vi "Fpga-Exercisor-Top.vi"() -> ()   [LabVIEW 2017]
uses:
  <vilib>/Platform/TimedLoop/XDataNode/timing_clust.ctl
  <vilib>/Platform/TimedLoop/XDataNode/nitl_modes.ctl
  <vilib>/Platform/TimedLoop/XDataNode/wakeup.ctl
  <vilib>/rvi/Emulation/niFpgaSctlEmulationGetInTimedLoop.vi
  <vilib>/rvi/Emulation/niFpgaEmulationReportErrorSimple.vi
  <vilib>/rvi/Emulation/niFpgaGetClockAttributes.vi
  <vilib>/rvi/Emulation/niFpgaCriticalErrorInLSC.vi
  <vilib>/rvi/eio/common/nirviEmuTemplateMethod_errors.vi
  <vilib>/rvi/interface/RandomDataEmulation/niFpgaRandomDataHandleErrors.vi
  <vilib>/Platform/TimedLoop/XDataNode/XDataNode.xnode
  <vilib>/eio/EIONode/EIONode.xnode
  <vilib>/rvi/DataTransferAndStorage/Container/XNode/niFpgaContainer.xnode
  <vilib>/rvi/interface/RandomDataEmulation/nirviRandomDataFpgaReadWriteTemplate.vi
  <vilib>/Platform/TimedLoop/XDataNode/XDNodeRunTimeDep.lvlib
panel:
  out "AXI_STR_RXD_tready 2":bool
  out "tvalid 2":bool
  out "tdata 2":u32
  out "tlast 2":bool
  out "AXI_STR_RXD_tready_Count 2":u16
  out "tvalid_Count 2":u16
  out "tlast_Count 2":u16
  out "tdata_LastNonZero 2":u32
  out "AXI_STR_RXD_tready":bool
  out "tvalid":bool
  out "tdata":u32
  out "tlast":bool
  out "AXI_STR_RXD_tready_Count":u16
  out "tvalid_Count":u16
  out "tlast_Count":u16
  out "tdata_LastNonZero":u32
  out "d_microblaze\\gpio2_out_tri_o":u32
  in  "d_microblaze\\gpio2_in_tri_i":u32
  out "d_microblaze\\gpio1_out_tri_o":u32
  in  "d_microblaze\\gpio1_in_tri_i":u32
  in  "d_microblaze\\Int_1":bool
  in  "d_microblaze\\Int_0":bool
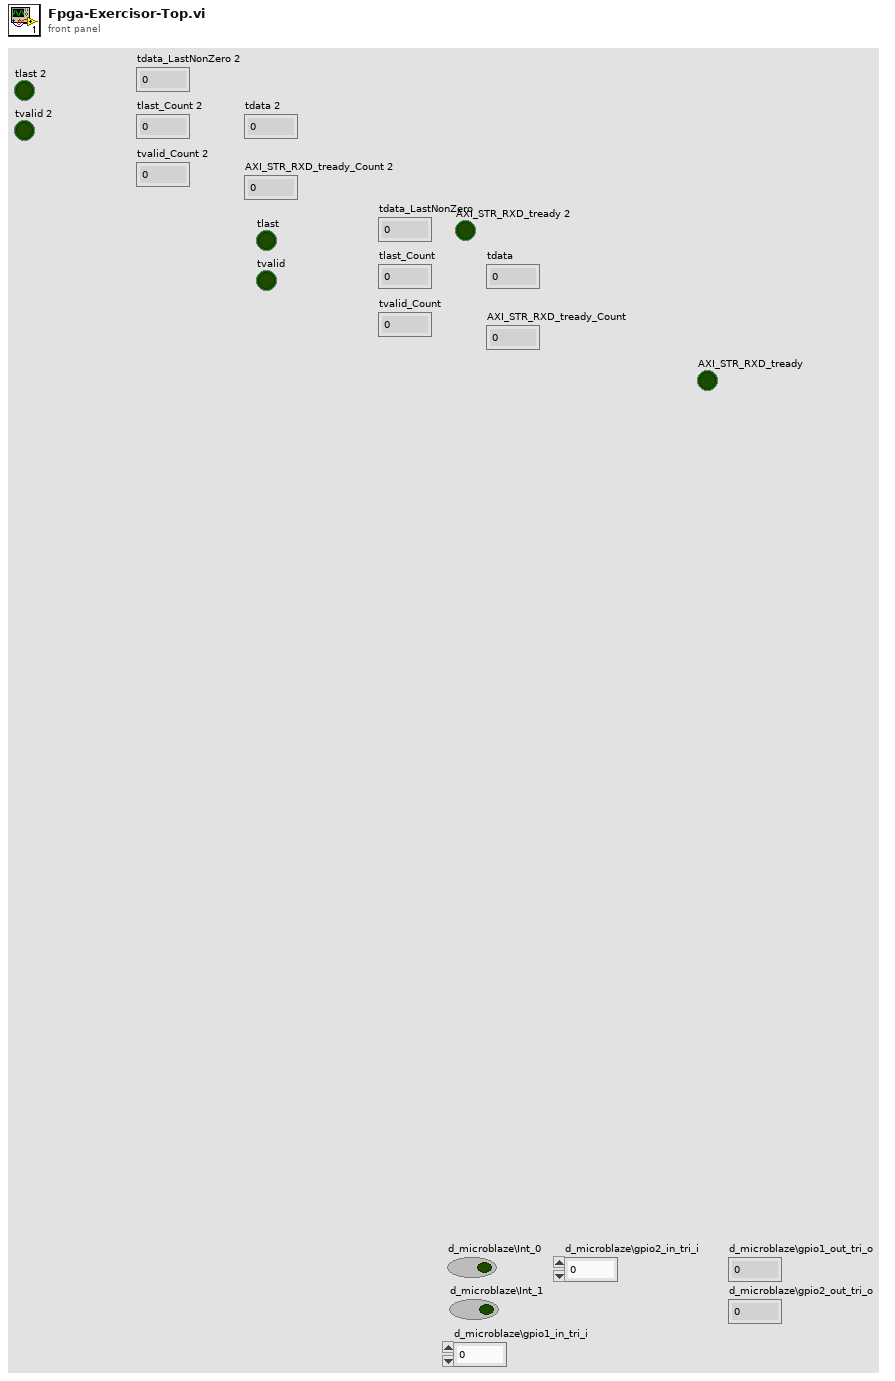
[diagram p1: front panel]
types:
  T1 = typedef "XDNodeRunTimeDep.lvlib/timing_clust.ctl" = cluster{"Expected End [f-1]":u64, "Actual End [f-1]":u64, "Finished Late? [f-1]":bool, "Expected End [i-1]":u64, "Actual End [i-1]":u64, "Finished Late? [i-1]":bool, "Expected Start [i]":u64, "Actual Start [i]":u64, "Expected Start [f]":u64, "Actual Start [f]":u64, "Source Name":string, "Structure Name":string, "Period":i64, "Deadline":i64, "Offset":i64, "Start":i64, "Priority":i32, "Timeout":i32, "Mode":T2, "Wakeup Reason":T3, "Error":errorcluster, "Source Type":string, "Secondary Source Type":string, "Global End Time":u64, "Global Start Time":u64, "Frame Duration":u64, "Iteration Duration":u64, "Assigned CPU":i32, "I/O Scan Engine Mode":u32}
  T2 = typedef "XDNodeRunTimeDep.lvlib/nitl_modes.ctl" = enum32{"No Change", "Process missed periods, maintain original phase", "Discard missed periods, maintain original phase", "Process missed periods, ignore original phase", "Discard missed periods, ignore original phase"}
  T3 = typedef "XDNodeRunTimeDep.lvlib/wakeup.ctl" = enum32{"Normal", "Aborted", "Asynchronous wakeup", "Timing source error", "Timed loop error", "Timeout"}
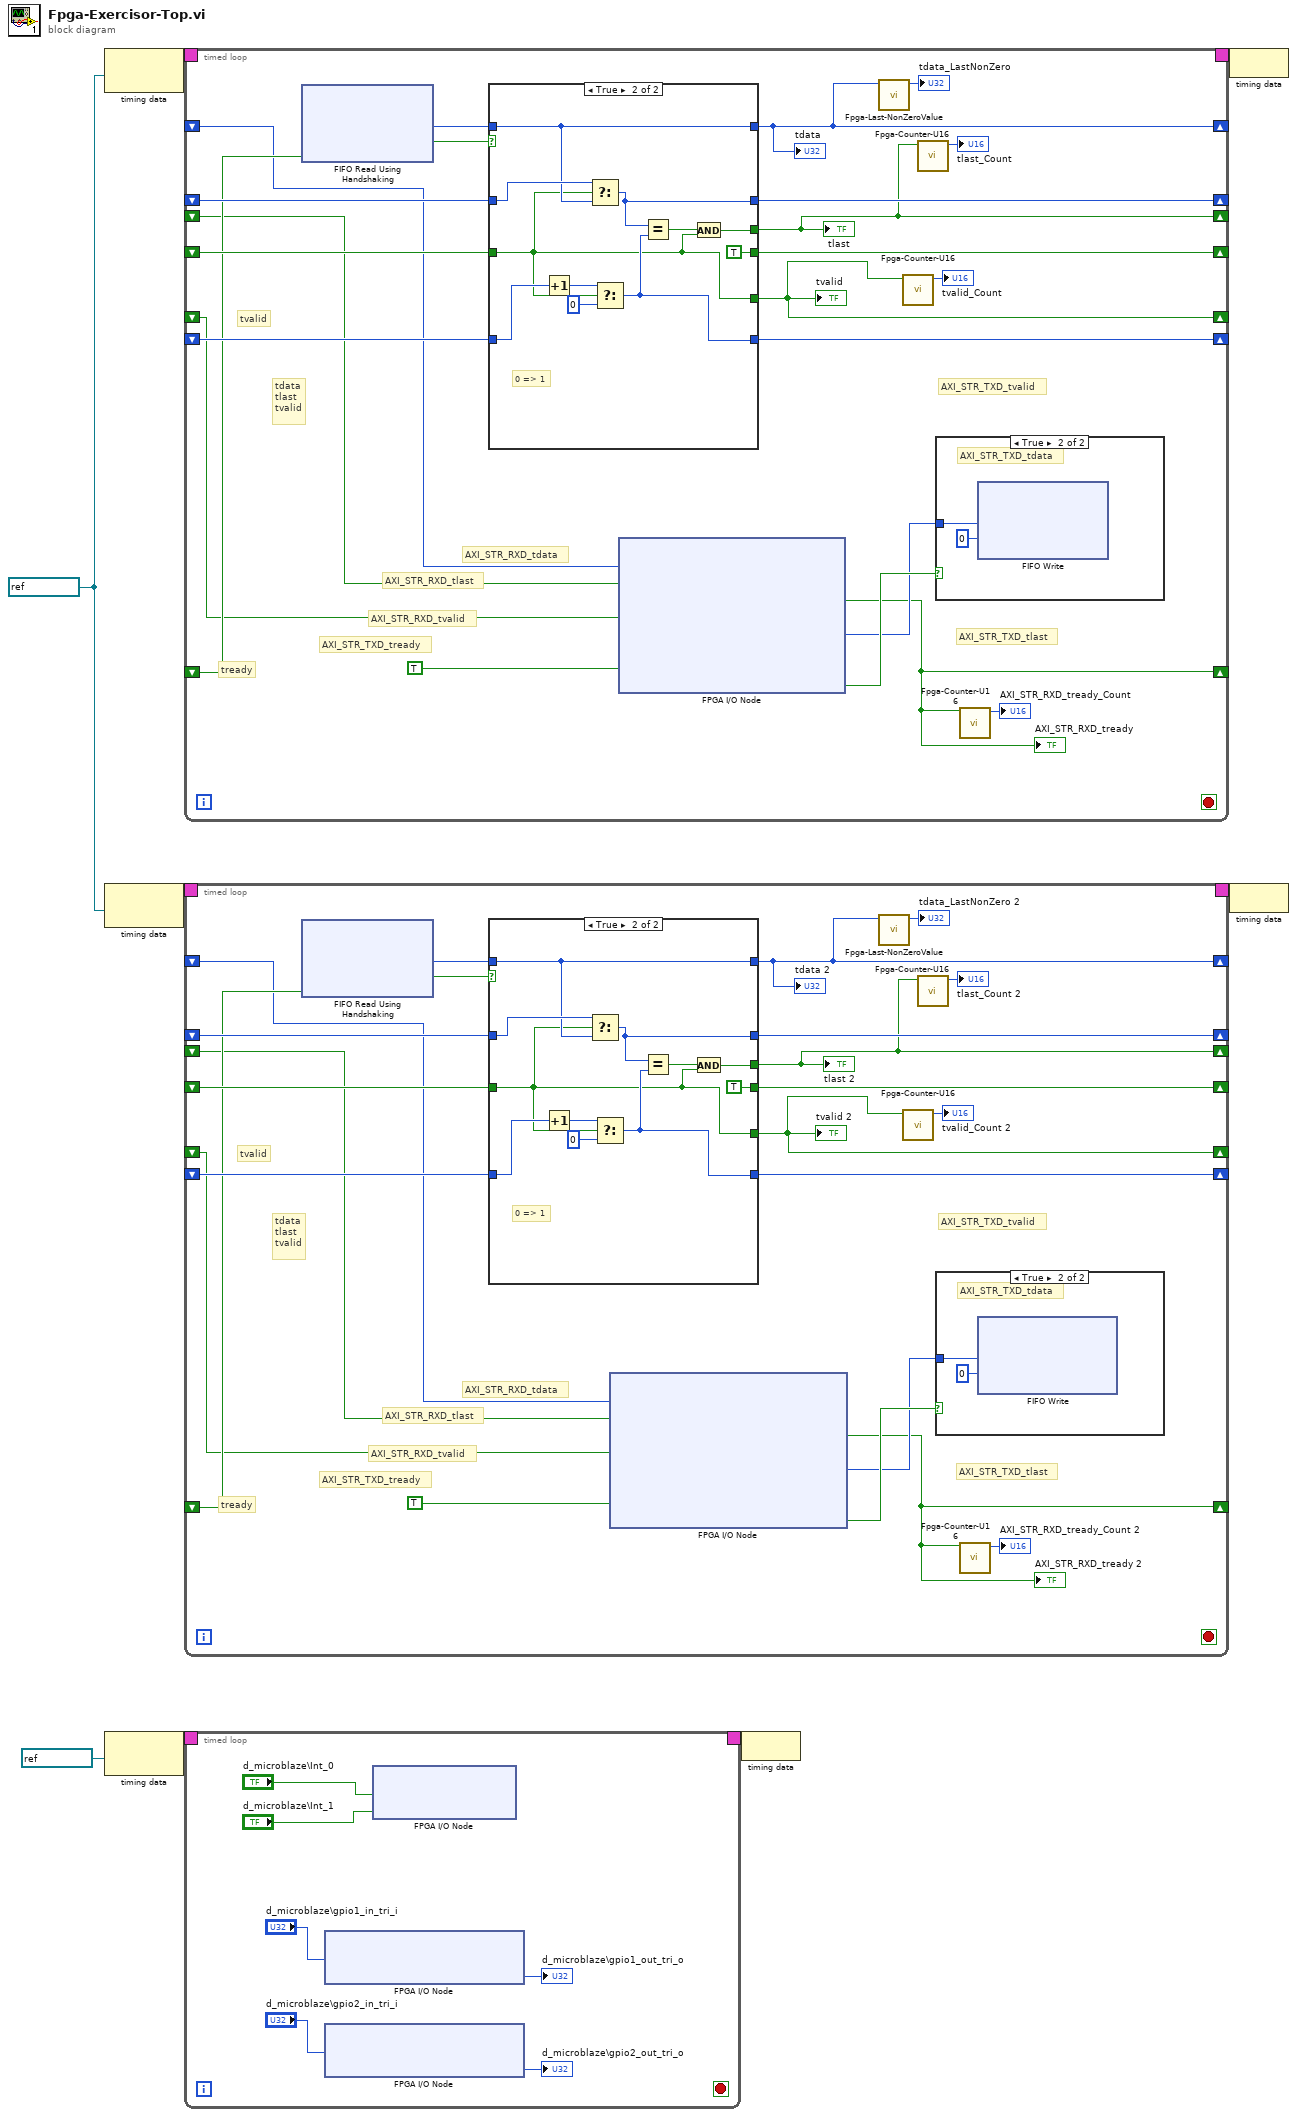
[diagram p0: block diagram]
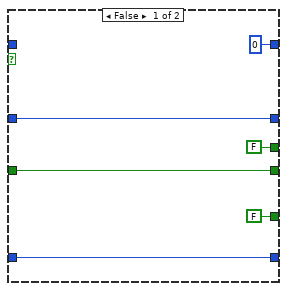
[diagram p3: hidden frame]
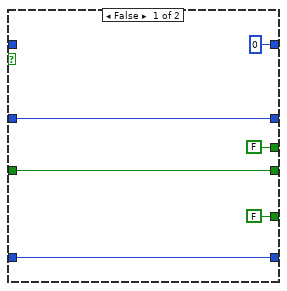
[diagram p5: hidden frame]
diagram:
  w1 = refnum<k21> "100MHz" ("Source Name")
  n1 = node-c288(w1) -> (w5:T1)
  n2 = node-c288(w1) -> (w3:T1)
  n3 = node-c288(refnum<k21> "100MHz" ("Source Name")) -> (w8:T1)
  n4 = timed-loop {
    timing: w5 -> [_]
    timing-out: [_] -> w4
    shift-right: [w29] -> _
    shift-left: _ -> [w30]
    shift-right: [w26] -> _
    shift-left: _ -> [w28]
    shift-right: [w24] -> _
    shift-left: _ -> [w25]
    shift-right: [w21] -> _
    shift-left: _ -> [w13]
    shift-right: [w9] -> _
    shift-left: _ -> [w23]
    shift-right: [w17] -> _
    shift-left: _ -> [w15]
    shift-right: [w19] -> _
    shift-left: _ -> [w14]
    stop <- _ stop-if-true
    # "AXI_STR_TXD_tlast"
    # "AXI_STR_TXD_tvalid"
    # "AXI_STR_TXD_tready"
    # "AXI_STR_RXD_tvalid"
    # "AXI_STR_RXD_tlast"
    # "AXI_STR_RXD_tdata"
    # "tvalid"
    # "tready"
    # "tdata\ntlast\ntvalid"
    n5 = xnode ("FIFO Read Using Handshaking")("Ready for Output"=w23) -> ("Element"=w27:u32, "Output Valid"=w31:bool)  [unwired: 1 in, 1 out]
    n6 = case shown="True" w31 {
      tunnel: w30 -> [w38 w40]
      tunnel: [w38 TRUE ("Size\nRead?")] -> w29
      tunnel: w28 -> [w39 w50]
      tunnel: w27 -> [_ w45]
      tunnel: [w39 w44] -> w26
      tunnel: w25 -> [w37 w49]
      tunnel: [w37 w43] -> w24
      tunnel: [FALSE ("Size\nRead?") w40] -> w21
      tunnel: [u32 0 ("Element") w45] -> w17
      tunnel: [FALSE w41] -> w19
      frame False {
      }
      frame True {
        # "0 => 1"
        n7 = Increment(x=w49) -> (x+1=w47:u32)
        n8 = Select(t=w50, s=w40, f=w45) -> (s? t:f=w44:u32)
        n9 = Select(t=w47, s=w40, f=u32 0) -> (s? t:f=w43:u32)
        n10 = Equal?(x=w44, y=w43) -> (x = y?=w42:bool)
        n11 = And(x=w42, y=w40) -> (x .and. y?=w41:bool)
      }
    }
    "tvalid" <- w21
    "tdata" <- w17
    "tlast" <- w19
    n12 = xnode "FPGA I/O Node"("d_microblaze\\AXI_STR_RXD_tdata"=w15, "d_microblaze\\AXI_STR_RXD_tlast"=w14, "d_microblaze\\AXI_STR_RXD_tvalid"=w13, "d_microblaze\\AXI_STR_TXD_tready"=TRUE ("d_microblaze\\AXI_STR_TXD_tready")) -> ("d_microblaze\\AXI_STR_RXD_tready"=w9:bool, "d_microblaze\\AXI_STR_TXD_tdata"=w10:u32, "d_microblaze\\AXI_STR_TXD_tvalid"=w11:bool)  [unwired: 8 in, 9 out]
    "AXI_STR_RXD_tready" <- w9
    n13 = call "Fpga-Last-NonZeroValue.vi"("d_mcs_i\\IO_BUS_write_data in"=w17) -> ("d_mcs_i\\IO_BUS_write_data out"=→"tdata_LastNonZero":u32)  [unwired: 10 in]
    n14 = call "Fpga-Counter-U16.vi"("d_mcs_i\\IO_BUS_read_strobe"=w21) -> ("Numeric"=→"tvalid_Count":u16)  [unwired: 10 in]
    n15 = call "Fpga-Counter-U16.vi"("d_mcs_i\\IO_BUS_read_strobe"=w19) -> ("Numeric"=→"tlast_Count":u16)  [unwired: 10 in]
    n16 = case shown="True" w11 {
      tunnel: w10 -> [_ w33]
      frame False {
      }
      frame True {
        # "AXI_STR_TXD_tdata"
        n17 = xnode ("FIFO Write")("Element"=w33, "Timeout"=0) -> ()  [unwired: 1 in, 2 out]
      }
    }
    n18 = call "Fpga-Counter-U16.vi"("d_mcs_i\\IO_BUS_read_strobe"=w9) -> ("Numeric"=→"AXI_STR_RXD_tready_Count":u16)  [unwired: 10 in]
  }
  n19 = timed-loop {
    timing: w3 -> [_]
    timing-out: [_] -> w2
    shift-right: [w73] -> _
    shift-left: _ -> [w74]
    shift-right: [w70] -> _
    shift-left: _ -> [w72]
    shift-right: [w68] -> _
    shift-left: _ -> [w69]
    shift-right: [w65] -> _
    shift-left: _ -> [w57]
    shift-right: [w53] -> _
    shift-left: _ -> [w67]
    shift-right: [w61] -> _
    shift-left: _ -> [w59]
    shift-right: [w63] -> _
    shift-left: _ -> [w58]
    stop <- _ stop-if-true
    # "AXI_STR_TXD_tlast"
    # "AXI_STR_TXD_tvalid"
    # "AXI_STR_TXD_tready"
    # "AXI_STR_RXD_tvalid"
    # "AXI_STR_RXD_tlast"
    # "AXI_STR_RXD_tdata"
    # "tvalid"
    # "tready"
    # "tdata\ntlast\ntvalid"
    n20 = xnode ("FIFO Read Using Handshaking")("Ready for Output"=w67) -> ("Element"=w71:u32, "Output Valid"=w75:bool)  [unwired: 1 in, 1 out]
    n21 = case shown="True" w75 {
      tunnel: w74 -> [w82 w84]
      tunnel: [w82 TRUE ("Size\nRead?")] -> w73
      tunnel: w72 -> [w83 w94]
      tunnel: w71 -> [_ w89]
      tunnel: [w83 w88] -> w70
      tunnel: w69 -> [w81 w93]
      tunnel: [w81 w87] -> w68
      tunnel: [FALSE ("Size\nRead?") w84] -> w65
      tunnel: [u32 0 ("Element") w89] -> w61
      tunnel: [FALSE w85] -> w63
      frame False {
      }
      frame True {
        # "0 => 1"
        n22 = Increment(x=w93) -> (x+1=w91:u32)
        n23 = Select(t=w94, s=w84, f=w89) -> (s? t:f=w88:u32)
        n24 = Select(t=w91, s=w84, f=u32 0) -> (s? t:f=w87:u32)
        n25 = Equal?(x=w88, y=w87) -> (x = y?=w86:bool)
        n26 = And(x=w86, y=w84) -> (x .and. y?=w85:bool)
      }
    }
    "tvalid 2" <- w65
    "tdata 2" <- w61
    "tlast 2" <- w63
    n27 = xnode "FPGA I/O Node"("d_microblaze\\AXI_STR_RXD_1_tdata"=w59, "d_microblaze\\AXI_STR_RXD_1_tlast"=w58, "d_microblaze\\AXI_STR_RXD_1_tvalid"=w57, "d_microblaze\\AXI_STR_TXD_1_tready"=TRUE ("d_microblaze\\AXI_STR_TXD_tready")) -> ("d_microblaze\\AXI_STR_RXD_1_tready"=w53:bool, "d_microblaze\\AXI_STR_TXD_1_tdata"=w54:u32, "d_microblaze\\AXI_STR_TXD_1_tvalid"=w55:bool)  [unwired: 8 in, 9 out]
    "AXI_STR_RXD_tready 2" <- w53
    n28 = call "Fpga-Last-NonZeroValue.vi"("d_mcs_i\\IO_BUS_write_data in"=w61) -> ("d_mcs_i\\IO_BUS_write_data out"=→"tdata_LastNonZero 2":u32)  [unwired: 10 in]
    n29 = call "Fpga-Counter-U16.vi"("d_mcs_i\\IO_BUS_read_strobe"=w65) -> ("Numeric"=→"tvalid_Count 2":u16)  [unwired: 10 in]
    n30 = call "Fpga-Counter-U16.vi"("d_mcs_i\\IO_BUS_read_strobe"=w63) -> ("Numeric"=→"tlast_Count 2":u16)  [unwired: 10 in]
    n31 = case shown="True" w55 {
      tunnel: w54 -> [_ w77]
      frame False {
      }
      frame True {
        # "AXI_STR_TXD_tdata"
        n32 = xnode ("FIFO Write")("Element"=w77, "Timeout"=0) -> ()  [unwired: 1 in, 2 out]
      }
    }
    n33 = call "Fpga-Counter-U16.vi"("d_mcs_i\\IO_BUS_read_strobe"=w53) -> ("Numeric"=→"AXI_STR_RXD_tready_Count 2":u16)  [unwired: 10 in]
  }
  n34 = timed-loop {
    timing: w8 -> [_]
    timing-out: [_] -> w7
    stop <- _ stop-if-true
    n35 = xnode "FPGA I/O Node"("d_microblaze\\gpio1_in_tri_i"="d_microblaze\\gpio1_in_tri_i") -> ("d_microblaze\\gpio1_out_tri_o"=→"d_microblaze\\gpio1_out_tri_o":u32)  [unwired: 2 in, 2 out]
    n36 = xnode "FPGA I/O Node"("d_microblaze\\gpio2_in_tri_i"="d_microblaze\\gpio2_in_tri_i") -> ("d_microblaze\\gpio2_out_tri_o"=→"d_microblaze\\gpio2_out_tri_o":u32)  [unwired: 2 in, 2 out]
    n37 = xnode "FPGA I/O Node"("d_microblaze\\Int_0"="d_microblaze\\Int_0", "d_microblaze\\Int_1"="d_microblaze\\Int_1") -> ()  [unwired: 2 in, 2 out]
  }
  n38 = node-c288(w7) -> ()
  n39 = node-c288(w4) -> ()
  n40 = node-c288(w2) -> ()
